vi "writestatus.vi"(10 "字符串":string) -> ()   [LabVIEW 2011]
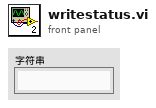
[diagram p1: front panel]
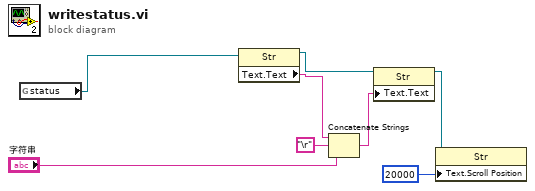
[diagram p0: block diagram]
diagram:
  n1 = global read "全局 1.vi" "status"() -> (w3:refnum<vi>)
  n2 = property on="属性节点" class="Str"(reference=w3) -> (reference out=w4:refnum<vi>, "Text.Text"=w6:string)  [unwired: 1 in, 1 out]
  n3 = Concatenate Strings(w6, "\r", "字符串") -> (w7:string)
  n4 = property on="属性节点" class="Str"(reference=w4, "Text.Text"=w7) -> (reference out=w2:refnum<vi>)  [unwired: 1 in, 1 out]
  n5 = property on="属性节点" class="Str"(reference=w2, "Text.Scroll Position"=u32 20000 ("文本.滚动条位置")) -> ()  [unwired: 1 in, 2 out]
